vi "Configure Hardware.vi"(8 "error in (no error)":errorcluster, 11 "Hardware Resources in":T1={"DAQmx Channel 1"="", "DAQmx Channel 2"="", "DAQmx Channel 3"="", "DAQmx AI Task"="", "Channel 1 Name"="Battery Voltage", "Channel 2 Name"="Battery Current", "Channel 3 Name"="Brake torque", "Sample time"=50, "Samples per second"=1000.0, "Sample mode"=10123, "Samples per channel"=0, "Offset Channel 1"=0.0, "Offset Channel 2"=0.0, "Offset Channel 3"=0.0, "Scale Channel 1"=0.0, "Scale Channel 2"=0.0, "Scale Channel 3"=0.0, "DAQmx Counter Channel"="", "Counter Name"="", "DAQmx Counter Task"=""} {"Sample mode" items=["Continuous Samples"=10123]}) -> (0 "error out":errorcluster, 3 "Hardware Resources out":T1={"DAQmx Channel 1"="", "DAQmx Channel 2"="", "DAQmx Channel 3"="", "DAQmx AI Task"="", "Channel 1 Name"="Battery Voltage", "Channel 2 Name"="Battery Current", "Channel 3 Name"="Brake torque", "Sample time"=50, "Samples per second"=1000.0, "Sample mode"=0, "Samples per channel"=0, "Offset Channel 1"=0.0, "Offset Channel 2"=0.0, "Offset Channel 3"=0.0, "Scale Channel 1"=0.0, "Scale Channel 2"=0.0, "Scale Channel 3"=0.0, "DAQmx Counter Channel"="", "Counter Name"="", "DAQmx Counter Task"=""} {"Sample mode" items=["Continuous Samples"=10123]})   [LabVIEW 2018, in "Acquisition.lvlib"]
doc: "Configure the hardware."
uses:
  Acquisition.lvlib
  Hardware Configuration.ctl
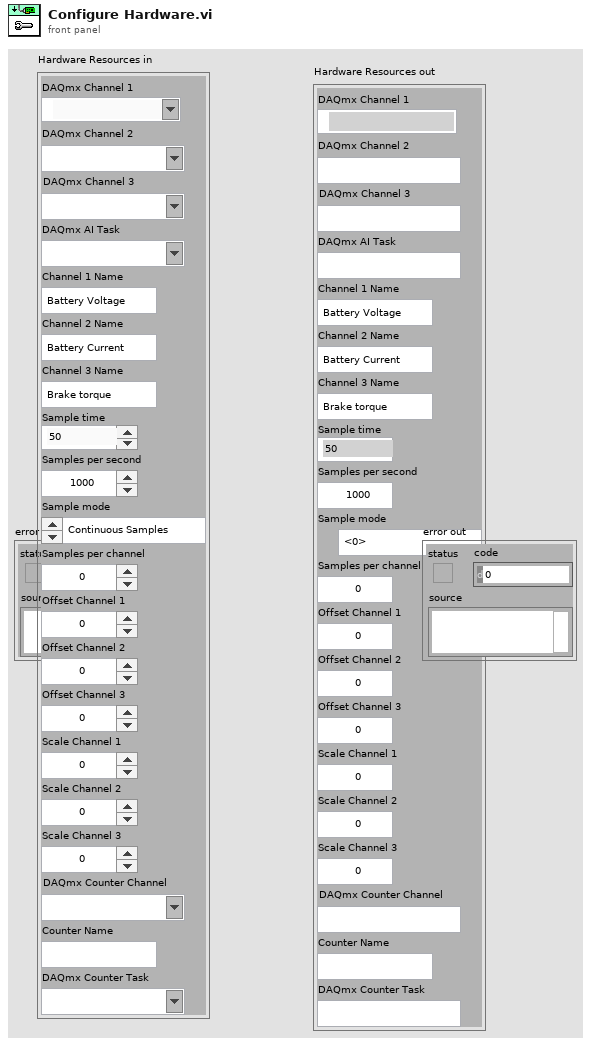
[diagram p1: front panel]
types:
  T1 = typedef "Acquisition.lvlib/Hardware Configuration.ctl" = cluster{"DAQmx Channel 1":tag, "DAQmx Channel 2":tag, "DAQmx Channel 3":tag, "DAQmx AI Task":refnum<k21>, "Channel 1 Name":string, "Channel 2 Name":string, "Channel 3 Name":string, "Sample time":u32, "Samples per second":dbl, "Sample mode":u16, "Samples per channel":i32, "Offset Channel 1":dbl, "Offset Channel 2":dbl, "Offset Channel 3":dbl, "Scale Channel 1":dbl, "Scale Channel 2":dbl, "Scale Channel 3":dbl, "DAQmx Counter Channel":tag, "Counter Name":string, "DAQmx Counter Task":refnum<k21>}
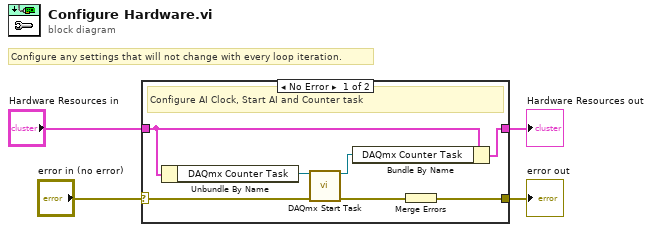
[diagram p0: block diagram]
diagram:
  # "Configure any settings that will not change with every loop iteration."
  n1 = case shown="No Error" "error in (no error)" {
    selector: "error in (no error)" -> [w8 w12]
    tunnel: [w7 w12] -> w3
    tunnel: "Hardware Resources in" -> [w10 w13]
    tunnel: [w11 w13] -> w1
    frame No Error {
      # "Configure AI Clock, Start AI and Counter task"
      n2 = Unbundle By Name(w10) -> ("DAQmx Counter Task"=w5:refnum<k21>)
      n3 = call <vilib>:"DAQmx Start Task.vi"("task/channels in"=w5, "error in"=w8) -> ("task out"=w9:refnum<k21>, "error out"=w6:errorcluster)  [unwired: 12 in]
      n4 = Bundle By Name(cluster=w10, "DAQmx Counter Task"=w9) -> (w11:T1)
      n5 = Merge Errors(w6) -> (w7:errorcluster)
    }
    frame Error {
    }
  }
  "Hardware Resources out" <- w1
  "error out" <- w3
